vi "SV TDMS Read Octave (1 Ch).vi"(0 "tdms file":refnum<k34>, 5 "group name in":string="Octave", 7 "channel name in":string="Channel0", 11 "error in":errorcluster) -> (3 "scale labels":T1, 4 "tdms file out":refnum<k34>, 6 "group name out":string, 8 "channel name out":string, 10 "octave spectrum":T2, 13 "octave info":T3={"standard"=enum."ANSI S1.11", "bandwidth"=enum."1 octave", "low band"=0, "high band"=0, "weighting filter"=0, "dB reference"=0.0, "dB On"=FALSE, "unit label"="", "channel name"="", "description"="", "engineering units"=1, "custom label"="", "spectrum type"=enum."magnitude", "spectral density"=FALSE, "filters settled"=FALSE} {"engineering units" items=["custom..."=0, "V"=1, "A"=21, "C"=30, "pC"=31, "s"=32, "-"=29, "Pa"=2, "N"=20, "g"=3, "m/s^2"=4, "m/s"=5, "m"=6, "mm/s"=12, "mm"=13, "micron/s"=14, "micron"=15, "in/s^2"=7, "in/s"=8, "in"=9, "mil/s"=10, "mil"=11, "rad/s^2"=16, "rad/s"=17, "rad"=18, "deg/s^2"=26, "deg/s"=27, "deg"=28, "RPM"=22, "cycle/s^2"=23, "Hz"=24, "cycle"=25, "strain"=19]; "dB reference" format="%.2e"; "weighting filter" items=["Linear", "A-weighting", "B-weighting", "C-weighting", "ITU-R 468-4", "Dolby", "CCITT", "C-message", "Wb", "Wc", "Wd", "We", "Wf", "Wh", "Wj", "Wk", "Wm", "AES17 20 kHz lowpass", "AES17 40 kHz lowpass", "AES17 20 kHz highpass", "AES17 40 kHz highpass"]}, 15 "error out":errorcluster)   [LabVIEW 2017]
doc: "Reads the specified .tdms file and returns data in a format specific to the polymorphic instance selected."
uses:
  <vilib>/addons/_NISVFA/_Shared subVIs/Controls/svc_Octave Info.ctl
  <vilib>/addons/_NISVFA/_Shared subVIs/Controls/svc_Octave Standard.ctl
  <vilib>/addons/_NISVFA/_Shared subVIs/Controls/svc_Weighting Filter Text Ring.ctl
  <vilib>/addons/_NISVFA/_Shared subVIs/Controls/svc_Engineering Units Text Ring.ctl
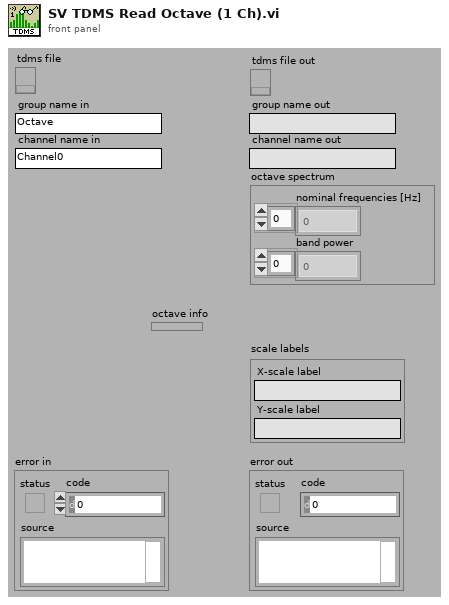
[diagram p1: front panel]
types:
  T1 = cluster{"X-scale label":string, "Y-scale label":string}
  T2 = cluster{"nominal frequencies [Hz]":dbl[], "band power":dbl[]}
  T3 = typedef "svc_Octave Info.ctl" = cluster{"standard":T4, "bandwidth":enum16{"1 octave", "1/3 octave", "1/6 octave", "1/12 octave", "1/24 octave"}, "low band":i32, "high band":i32, "weighting filter":T5, "dB reference":dbl, "dB On":bool, "unit label":string, "channel name":string, "description":string, "engineering units":T6, "custom label":string, "spectrum type":enum16{"power", "magnitude"}, "spectral density":bool, "filters settled":bool}
  T4 = typedef "svc_Octave Standard.ctl" = enum16{"ANSI S1.11", "IEC 61260"}
  T5 = typedef "svc_Weighting Filter Text Ring.ctl" = u16
  T6 = typedef "svc_Engineering Units Text Ring.ctl" = u16
  T7 = cluster{"nominal frequencies [Hz]":dbl[], "nominal frequencies [Hz]":dbl[]}
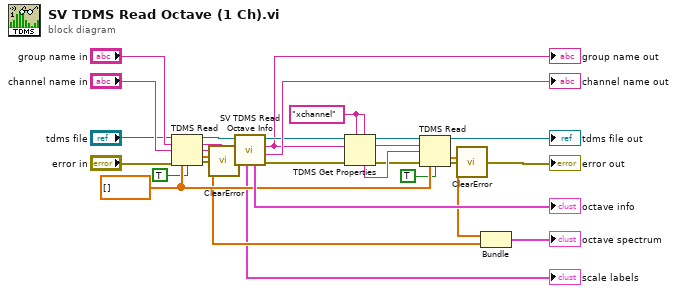
[diagram p0: block diagram]
diagram:
  w22 = dbl[] [] ("nominal frequencies [Hz]")
  w12 = "xchannel" ("channel name")
  n1 = TDMS Read(0:"tdms file", 5:"group name in", 7:"channel name in", 11:"error in", 12:w22, 13:TRUE ("return channels in file order? (F)")) -> (4:w28:refnum<k34>, 6:w27:string, 8:w29:string, 10:w19:dbl[], 15:w4:errorcluster)  [unwired: 2 in, 1 out]
  n2 = call <vilib>:"ClearError.vi"("error in (no error)"=w4) -> ("error out"=w26:errorcluster)
  n3 = call <vilib>:"SV TDMS Read Octave Info.vi"("error in"=w26, "channel name in"=w29, "group name in"=w27, "tdms file"=w28) -> ("error out"=w14:errorcluster, "channel name out"=→"channel name out":string, "group name out"=w13:string, "tdms file out"=w15:refnum<k34>, "octave info"=→"octave info":T3, "labels"=→"scale labels":T1)  [unwired: 2 in]
  "group name out" <- w13
  n4 = TDMS Get Properties(5:w12, 7:w12, 8:w14, 10:w13, 11:w15) -> (0:w8:errorcluster, 2:w10:string, 3:w11:refnum<k34>, 4:w9:string)  [unwired: 1 in, 2 out]
  n5 = TDMS Read(0:w11, 5:w10, 7:w9, 11:w8, 12:w22, 13:TRUE ("return channels in file order? (F)")) -> (4:→"tdms file out":refnum<k34>, 10:w21:dbl[], 15:w3:errorcluster)  [unwired: 2 in, 3 out]
  n6 = call <vilib>:"ClearError.vi"("error in (no error)"=w3) -> ("error out"=→"error out":errorcluster)
  n7 = Bundle("nominal frequencies [Hz]"=w21, "nominal frequencies [Hz]"=w19) -> (→"octave spectrum":T7)  [unwired: 1 in]
